vi "GPIB.vi"() -> ()   [LabVIEW 2017]
panel:
  in  "タイムアウト":u32=10
  out "受信文字列":string
  in  "終了ボタン":bool
  in  "ボードID":string="0"
  in  "機器アドレス":string="1"
  in  "コマンド":string="*IDN?"
  in  "送受信ボタン":bool
  in  "クリアボタン":bool
  # "秒"
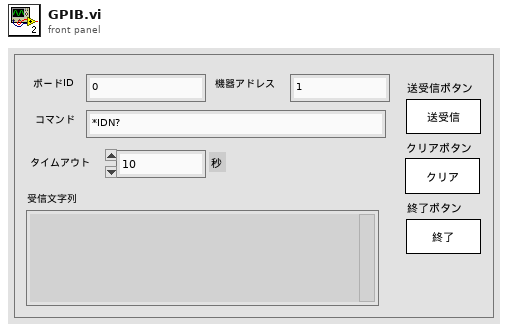
[diagram p1: front panel]
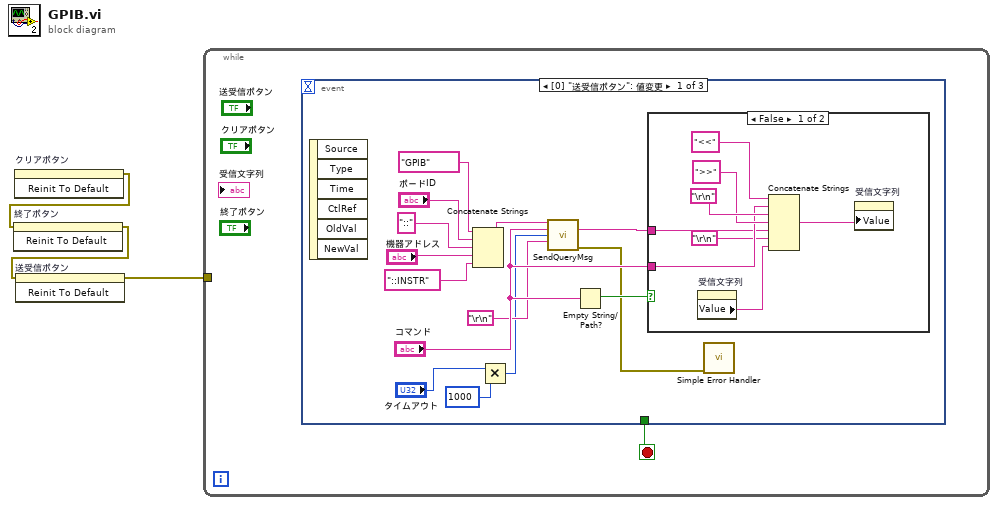
[diagram p0: block diagram]
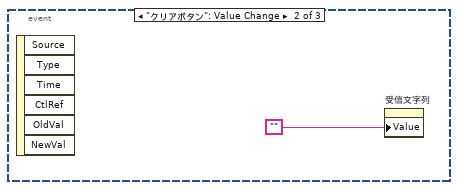
[diagram p3: hidden frame]
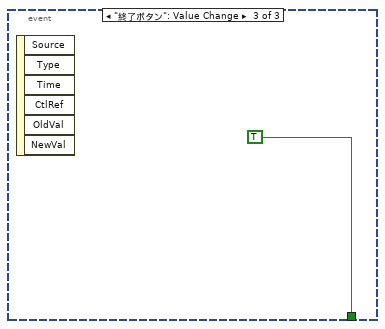
[diagram p4: hidden frame]
diagram:
  n1 = invoke on="クリアボタン" class="Bool" method="Reinit To Default"() -> (error out=w3:errorcluster)  [unwired: 3 in, 2 out]
  n2 = invoke on="終了ボタン" class="Bool" method="Reinit To Default"(error in=w3) -> (error out=w2:errorcluster)  [unwired: 2 in, 2 out]
  n3 = invoke on="送受信ボタン" class="Bool" method="Reinit To Default"(error in=w2) -> (error out=w1:errorcluster)  [unwired: 2 in, 2 out]
  n4 = while {
    tunnel: w1 -> [_]
    stop <- w4 stop-if-true
    n5 = event shown="[0] \"送受信ボタン\": 値変更" {
      selector: _ -> [_ _ _]
      dyn-events: _ -> [_ _ _]
      timeout: _ -> [_ _ _]
      tunnel: [_ _ TRUE] -> w4
      event "送受信ボタン": Value Change {
        n6 = event-data() -> ()  [unwired: 1 in, 6 out]
        n7 = Concatenate Strings("GPIB", "ボードID", "::", "機器アドレス", "::INSTR") -> (w12:string)
        n8 = Multiply(x="タイムアウト", y=u32 1000 ("x")) -> (x*y=w6:u32)
        n9 = call "SendQueryMsg.vi"("VISAリソース名"=w12, "入力文字列"="コマンド", "タイムアウト"=w6, "ターミネータ"="\r\n") -> ("受信文字列"=w9:string, "エラー出力"=w10:errorcluster)  [unwired: 10 in]
        n10 = Empty String/Path?(string/path="コマンド") -> (empty?=w13:bool)
        n11 = case shown="FALSE" w13 {
          tunnel: "コマンド" -> [w23 _]
          tunnel: w9 -> [w22 _]
          frame False {
            n12 = property on="受信文字列" class="Str"() -> ("Value"=w19:string)  [unwired: 2 in, 2 out]
            n13 = Concatenate Strings("<<", w23, "\r\n", ">>", w22, "\r\n", w19) -> (w21:string)
            n14 = property on="受信文字列" class="Str"("Value"=w21) -> ()  [unwired: 2 in, 2 out]
          }
          frame True {
          }
        }
        n15 = call <vilib>:"Simple Error Handler.vi"("error in (no error)"=w10) -> ()  [unwired: 4 in, 5 out]
      }
      event "クリアボタン": Value Change {
        n16 = event-data() -> ()  [unwired: 1 in, 6 out]
        n17 = property on="受信文字列" class="Str"("Value"="") -> ()  [unwired: 2 in, 2 out]
      }
      event "終了ボタン": Value Change {
        n18 = event-data() -> ()  [unwired: 1 in, 6 out]
      }
    }
  }
